vi "HVSMeasurementGFV.vi"(8 "error in (no error)":errorcluster, 10 "Variant in":variant, 11 "HVSenum":T1=enum."InsertMeasurement") -> (0 "error out":errorcluster, 3 "Variant out":variant)   [LabVIEW 2013]
doc: "Use this template to build a VI to use as a subVI."
uses:
  HVSmeasurementEnum.ctl
  HVSmeasurementCluster.ctl
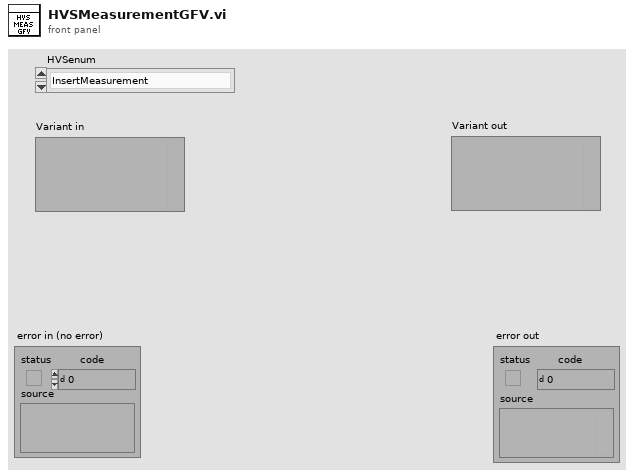
[diagram p1: front panel]
types:
  T1 = typedef "HVSmeasurementEnum.ctl" = enum16{"SaveRawDataToFile", "GetRunTime", "GetDataString", "Get WindSpeedDirectionVsTime", "Get TotalVolumeAndRuntimeVsTime", "Get PressureTempVsTime", "InsertMeasurement", "Init"}
  T2 = typedef "HVSmeasurementCluster.ctl" = cluster{"Time Stamp":timestamp, "Ambient Pressure (mbar)":dbl, "Temperature (Celcius)":dbl, "Wind Speed (m/s)":dbl, "Wind Direction (deg)":dbl, "Total Volume(m^3)":dbl, "Corrected Total Volume (m^3)":dbl, "RunTime (Min)":dbl}
  T3 = enum16{"open", "replace", "create", "open or create", "replace or create", "replace or create with confirmation"}
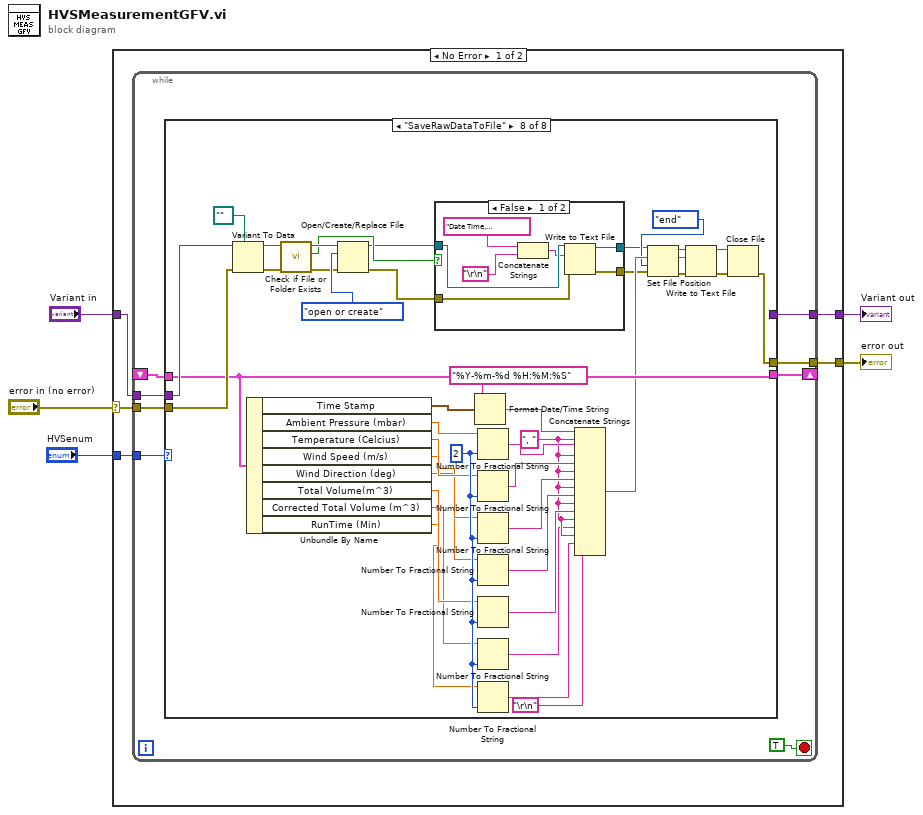
[diagram p0: block diagram]
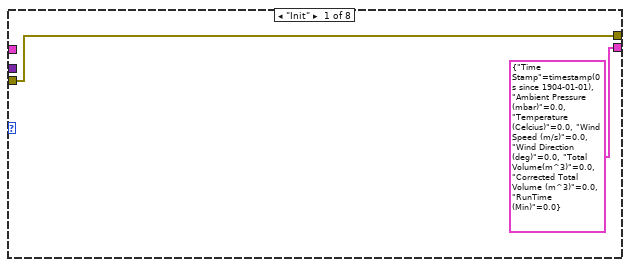
[diagram p2: hidden frame]
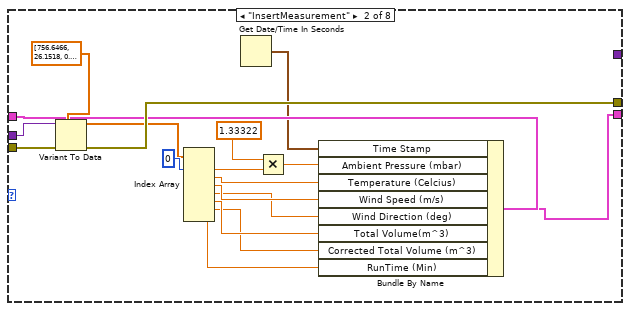
[diagram p3: hidden frame]
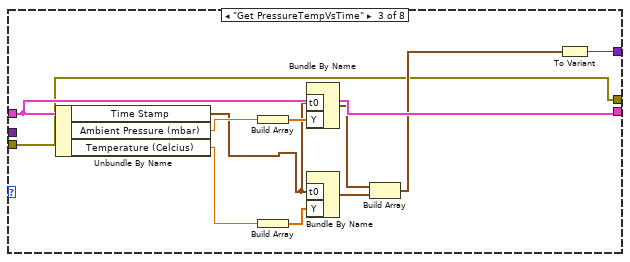
[diagram p4: hidden frame]
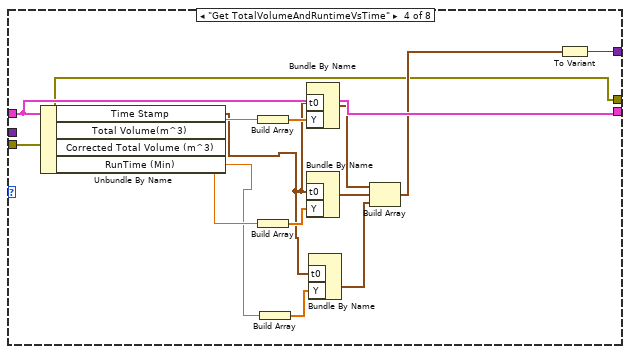
[diagram p5: hidden frame]
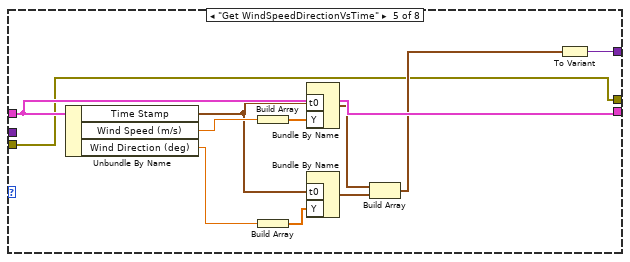
[diagram p6: hidden frame]
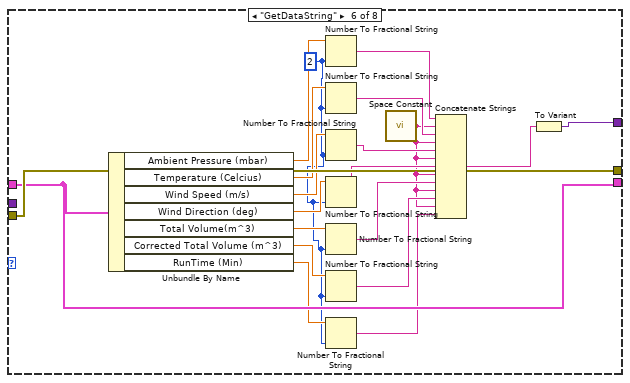
[diagram p7: hidden frame]
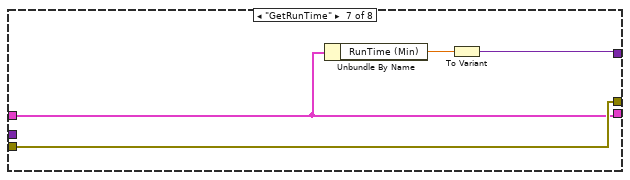
[diagram p8: hidden frame]
diagram:
  n1 = case shown="No Error" "error in (no error)" {
    selector: "error in (no error)" -> [w8 w150]
    tunnel: [w7 w150] -> w4
    tunnel: "HVSenum" -> [w10 _]
    tunnel: "Variant in" -> [w9 w149]
    tunnel: [w6 w149] -> w2
    frame No Error {
      n2 = while {
        tunnel: w10 -> [w17]
        shift-right: [w16] -> _
        shift-left: _ -> [w15]
        tunnel: w9 -> [w14]
        tunnel: w8 -> [w13]
        tunnel: [w12] -> w7
        tunnel: [w11] -> w6
        stop <- TRUE stop-if-true
        n3 = case shown="\"SaveRawDataToFile\"" w17 {
          tunnel: [T2 {"Time Stamp"=timestamp(0 s since 1904-01-01), "Ambient Pressure (mbar)"=0.0, "Temperature (Celcius)"=0.0, "Wind Speed (m/s)"=0.0, "Wind Direction (deg)"=0.0, "Total Volume(m^3)"=0.0, "Corrected Total Volume (m^3)"=0.0, "RunTime (Min)"=0.0} w29 w49 w63 w74 w93 w97 w128] -> w16
          tunnel: w15 -> [_ w30 w49 w63 w74 w93 w97 w128]
          tunnel: w14 -> [_ w37 _ _ _ _ _ w136]
          tunnel: w13 -> [w20 w38 w39 w54 w64 w94 w98 w135]
          tunnel: [w20 w36 w39 w54 w64 w94 w98 w105] -> w12
          tunnel: [_ _ w41 w56 w66 w76 w95 _] -> w11
          frame "Init" {
          }
          frame "InsertMeasurement" {
            n4 = Variant To Data(error in=w38, type=dbl[] [756.6466, 26.1518, 0.0, 0.0, 13023.23, 12973.74, 11564.0] ("HVS Data Array"), Variant=w37) -> (data=w31:dbl[], error out=w36:errorcluster)
            n5 = Index Array(array=w31, index #1=0 ("index")) -> (element #1=w32:dbl, element #2=w27:dbl, element #3=w26:dbl, element #4=w25:dbl, element #5=w24:dbl, element #6=w23:dbl, element #7=w22:dbl)  [unwired: 6 in]
            n6 = Get Date/Time In Seconds() -> (seconds since 1Jan1904=w21:timestamp)
            n7 = Multiply(x=1.33322, y=w32) -> (x*y=w28:dbl)
            n8 = Bundle By Name(cluster=w30, "Time Stamp"=w21, "Ambient Pressure (mbar)"=w28, "Temperature (Celcius)"=w27, "Wind Speed (m/s)"=w26, "Wind Direction (deg)"=w25, "Total Volume(m^3)"=w24, "Corrected Total Volume (m^3)"=w23, "RunTime (Min)"=w22) -> (w29:T2)
          }
          frame "Get PressureTempVsTime" {
            n9 = Unbundle By Name(w49) -> ("Time Stamp"=w42:timestamp, "Ambient Pressure (mbar)"=w44:dbl, "Temperature (Celcius)"=w43:dbl)
            n10 = Build Array(w44) -> (w48:dbl[])
            n11 = Build Array(w43) -> (w46:dbl[])
            n12 = Bundle By Name("t0"=w42, "Y"=w48) -> (w47:waveform(dbl))  [unwired: 1 in]
            n13 = Bundle By Name("t0"=w42, "Y"=w46) -> (w45:waveform(dbl))  [unwired: 1 in]
            n14 = Build Array(w47, w45) -> (w40:waveform(dbl)[])
            n15 = To Variant(anything=w40) -> (Variant=w41:variant)
          }
          frame "Get TotalVolumeAndRuntimeVsTime" {
            n16 = Unbundle By Name(w63) -> ("Time Stamp"=w52:timestamp, "Total Volume(m^3)"=w58:dbl, "Corrected Total Volume (m^3)"=w57:dbl, "RunTime (Min)"=w51:dbl)
            n17 = Build Array(w58) -> (w62:dbl[])
            n18 = Build Array(w57) -> (w60:dbl[])
            n19 = Build Array(w51) -> (w53:dbl[])
            n20 = Bundle By Name("t0"=w52, "Y"=w62) -> (w61:waveform(dbl))  [unwired: 1 in]
            n21 = Bundle By Name("t0"=w52, "Y"=w60) -> (w59:waveform(dbl))  [unwired: 1 in]
            n22 = Bundle By Name("t0"=w52, "Y"=w53) -> (w50:waveform(dbl))  [unwired: 1 in]
            n23 = Build Array(w61, w59, w50) -> (w55:waveform(dbl)[])
            n24 = To Variant(anything=w55) -> (Variant=w56:variant)
          }
          frame "Get WindSpeedDirectionVsTime" {
            n25 = Unbundle By Name(w74) -> ("Time Stamp"=w67:timestamp, "Wind Speed (m/s)"=w69:dbl, "Wind Direction (deg)"=w68:dbl)
            n26 = Build Array(w69) -> (w73:dbl[])
            n27 = Build Array(w68) -> (w71:dbl[])
            n28 = Bundle By Name("t0"=w67, "Y"=w73) -> (w72:waveform(dbl))  [unwired: 1 in]
            n29 = Bundle By Name("t0"=w67, "Y"=w71) -> (w70:waveform(dbl))  [unwired: 1 in]
            n30 = Build Array(w72, w70) -> (w65:waveform(dbl)[])
            n31 = To Variant(anything=w65) -> (Variant=w66:variant)
          }
          frame "GetDataString" {
            w75 = i16 2 ("precision (6)")
            n32 = Unbundle By Name(w93) -> ("Ambient Pressure (mbar)"=w92:dbl, "Temperature (Celcius)"=w91:dbl, "Wind Speed (m/s)"=w90:dbl, "Wind Direction (deg)"=w89:dbl, "Total Volume(m^3)"=w88:dbl, "Corrected Total Volume (m^3)"=w87:dbl, "RunTime (Min)"=w86:dbl)
            n33 = Number To Fractional String(number=w92, precision (6)=w75) -> (F-format string=w85:string)  [unwired: 2 in]
            n34 = Number To Fractional String(number=w91, precision (6)=w75) -> (F-format string=w84:string)  [unwired: 2 in]
            n35 = Number To Fractional String(number=w90, precision (6)=w75) -> (F-format string=w83:string)  [unwired: 2 in]
            n36 = Number To Fractional String(number=w89, precision (6)=w75) -> (F-format string=w82:string)  [unwired: 2 in]
            n37 = Number To Fractional String(number=w88, precision (6)=w75) -> (F-format string=w81:string)  [unwired: 2 in]
            n38 = Number To Fractional String(number=w87, precision (6)=w75) -> (F-format string=w80:string)  [unwired: 2 in]
            n39 = Number To Fractional String(number=w86, precision (6)=w75) -> (F-format string=w78:string)  [unwired: 2 in]
            n40 = call <vilib>:"Space Constant.vi"() -> ("String"=w79:string)
            n41 = Concatenate Strings(w85, w79, w84, w79, w83, w79, w82, w79, w81, w79, w80, w79, w78) -> (w77:string)
            n42 = To Variant(anything=w77) -> (Variant=w76:variant)
          }
          frame "GetRunTime" {
            n43 = Unbundle By Name(w97) -> ("RunTime (Min)"=w96:dbl)
            n44 = To Variant(anything=w96) -> (Variant=w95:variant)
          }
          frame "SaveRawDataToFile" {
            w124 = i16 2 ("precision (6)")
            w111 = ", " ("string")
            n45 = Variant To Data(error in=w135, type=path "" ("GRIMM File Path"), Variant=w136) -> (data=w139:path, error out=w138:errorcluster)
            n46 = Unbundle By Name(w128) -> ("Time Stamp"=w126:timestamp, "Ambient Pressure (mbar)"=w123:dbl, "Temperature (Celcius)"=w122:dbl, "Wind Speed (m/s)"=w121:dbl, "Wind Direction (deg)"=w120:dbl, "Total Volume(m^3)"=w119:dbl, "Corrected Total Volume (m^3)"=w118:dbl, "RunTime (Min)"=w117:dbl)
            n47 = call <vilib>:"Check if File or Folder Exists.vi"("error in (no error)"=w138, "path"=w139) -> ("error out"=w133:errorcluster, "file or folder exists?"=w131:bool, "dup path"=w132:path)  [unwired: 7 in]
            n48 = Open/Create/Replace File(file path (use dialog)=w132, error in=w133, operation (0:open)=T3."open or create") -> (refnum out=w130:refnum<file>, error out=w129:errorcluster)  [unwired: 3 in, 1 out]
            n49 = case shown="False" w131 {
              tunnel: w130 -> [w144 w148]
              tunnel: w129 -> [w142 w147]
              tunnel: [w141 w147] -> w102
              tunnel: [w140 w148] -> w100
              frame False {
                n50 = Concatenate Strings("Date Time, Pressure(mbar), Temp(deg), Wind Speed(m/s), Wind direction(deg), Total Vol (m^3), Corrected Total Vol (m^3), Run time(min)" ("string"), "\r\n") -> (w143:string)
                n51 = Write to Text File(file (use dialog)=w144, text=w143, error in=w142) -> (refnum out=w140:refnum<file>, error out=w141:errorcluster)  [unwired: 1 in, 1 out]
              }
              frame True {
              }
            }
            n52 = Format Date/Time String(time format string (%c)="%Y-%m-%d %H:%M:%S", seconds (now)=w126) -> (date/time string=w125:string)  [unwired: 1 in]
            n53 = Number To Fractional String(number=w123, precision (6)=w124) -> (F-format string=w116:string)  [unwired: 2 in]
            n54 = Number To Fractional String(number=w122, precision (6)=w124) -> (F-format string=w115:string)  [unwired: 2 in]
            n55 = Number To Fractional String(number=w121, precision (6)=w124) -> (F-format string=w114:string)  [unwired: 2 in]
            n56 = Number To Fractional String(number=w120, precision (6)=w124) -> (F-format string=w113:string)  [unwired: 2 in]
            n57 = Number To Fractional String(number=w119, precision (6)=w124) -> (F-format string=w112:string)  [unwired: 2 in]
            n58 = Number To Fractional String(number=w118, precision (6)=w124) -> (F-format string=w110:string)  [unwired: 2 in]
            n59 = Number To Fractional String(number=w117, precision (6)=w124) -> (F-format string=w109:string)  [unwired: 2 in]
            n60 = Concatenate Strings(w125, w111, w116, w111, w115, w111, w114, w111, w113, w111, w112, w111, w110, w111, w109, "\r\n") -> (w108:string)
            n61 = Set File Position(refnum=w100, from (0:start)=enum16{"start", "end", "current"}."end", error in=w102) -> (refnum out=w99:refnum<file>, error out=w101:errorcluster)  [unwired: 1 in]
            n62 = Write to Text File(file (use dialog)=w99, text=w108, error in=w101) -> (refnum out=w107:refnum<file>, error out=w106:errorcluster)  [unwired: 1 in, 1 out]
            n63 = Close File(refnum=w107, error in=w106) -> (error out=w105:errorcluster)  [unwired: 1 out]
          }
        }
      }
    }
    frame Error {
    }
  }
  "error out" <- w4
  "Variant out" <- w2
